vi "PV Pumping station controlling.vi"(8 "error in (no error)":errorcluster, 9 "PV Pumping station - Cluster":T1={"Parameter"=0, "Parameter\nread only<->describe"=FALSE, "Op. mode backing pump"=0, "Pmin for backing-pump\ninterval operations [W]"=40, "Config. Acces. A1 (old version)"=0, "Config. Acces. B1 (old version)"=0, "Pmax for backing-pump\ninterval operations [W]"=40} {"Pmax for backing-pump\ninterval operations [W]" min=30 max=90 step=1; "Config. Acces. B1 (old version)" items=[" fan (constant) (default)", " venting valve", " heating", " backing pump", " fan (temperature controlled)", " seal gas", " always off", " always on"]; "Config. Acces. A1 (old version)" items=[" fan (constant)", " venting valve", " heating", " backing pump", " fan (temperature controlled)", " seal gas", " always off", " always on"]; "Op. mode backing pump" items=[" non-stop", " intermittent", " switch on delayed"]; "Pmin for backing-pump\ninterval operations [W]" min=30 max=90 step=1; "Parameter" items=[" Operations mode backing pump (default)", " Configuration Accessories A1 (old version)", " Configuration Accessories B1 (old version)", " Actual pressure value  [mbar]   (read only)", " Vacuum pressure gauge type", " Pmin for backing-pump interval operations [W]", " Pmax for backing-pump interval operations [W]"]}, 10 "Adress of unit":u16=1 min=1 max=999 step=1, 11 "VISA session":refnum<visa-resource-name>) -> (0 "error out":errorcluster, 2 "response (data)":string, 3 "dup VISA session":refnum<visa-resource-name>)   [LabVIEW 2016, in "Pfeiffer Vacuum.lvlib"]
doc: "There are 7 parameters available, only one of which can be enabled at a time. \n\n0 - Operations mode backing pump (default) (025)\n1 - Configuration Accessories A1 (035)\n (old version - new in PV config A D input output.vi)\n2 - Configuration Accessories B1 (036)\n (old version - new in PV config A D input output.vi)\n3 - Actual pressure value [mbar] (read only) (340)\n4 - Vacuum pressure gauge type (738)\n5 - Pmin for backing-pump interval operations [W] (710)\n6 - Pmax for backing-pump interval operations [W] (711)\n\nNote: Any settings for an parameter that is not selected will be ignored. If a value is out of range, it will be changed to either the upper or the lower limit of the range."
uses:
  Pfeiffer Vacuum.lvlib
  PV Pumping station - Cluster.ctl
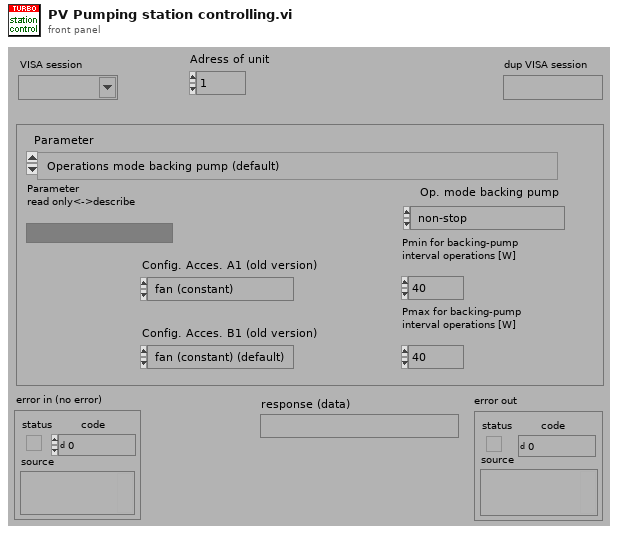
[diagram p1: front panel]
types:
  T1 = typedef "Pfeiffer Vacuum.lvlib/PV Pumping station - Cluster.ctl" = cluster{"Parameter":u16, "Parameter\nread only<->describe":bool, "Op. mode backing pump":u16, "Pmin for backing-pump\ninterval operations [W]":u16, "Config. Acces. A1 (old version)":u16, "Config. Acces. B1 (old version)":u16, "Pmax for backing-pump\ninterval operations [W]":u16}
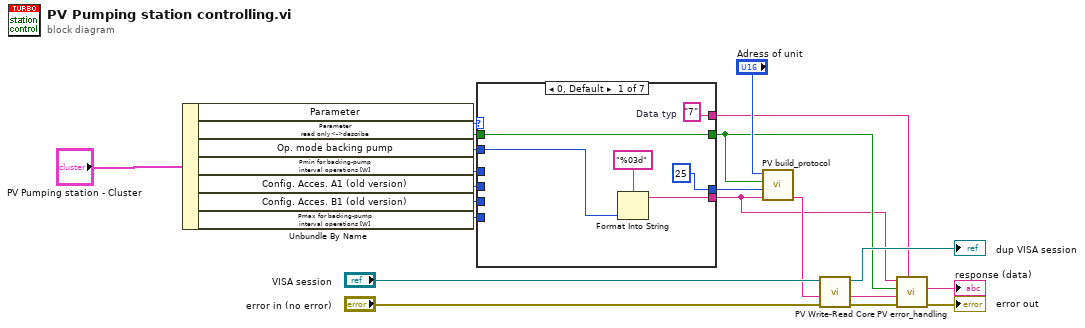
[diagram p0: block diagram]
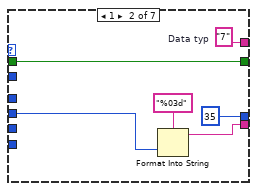
[diagram p2: hidden frame]
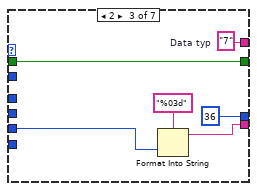
[diagram p3: hidden frame]
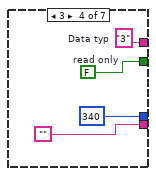
[diagram p4: hidden frame]
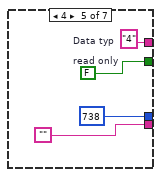
[diagram p5: hidden frame]
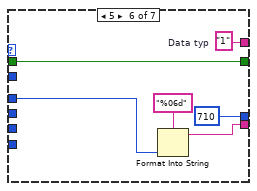
[diagram p6: hidden frame]
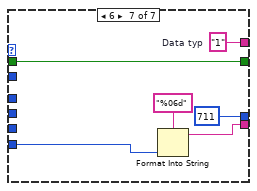
[diagram p7: hidden frame]
diagram:
  n1 = Unbundle By Name("PV Pumping station - Cluster") -> ("Parameter"=w19:u16, "Parameter\nread only<->describe"=w18:bool, "Op. mode backing pump"=w2:u16, "Pmin for backing-pump\ninterval operations [W]"=w14:u16, "Config. Acces. A1 (old version)"=w17:u16, "Config. Acces. B1 (old version)"=w16:u16, "Pmax for backing-pump\ninterval operations [W]"=w15:u16)
  n2 = case shown="0, Default" w19 {
    tunnel: [u16 25 ("Parameter-number") u16 35 ("Parameter-number") u16 36 ("Parameter-number") u16 340 ("Parameter-number") u16 738 ("Parameter-number") u16 710 ("Parameter-number") u16 711 ("Parameter-number")] -> w20
    tunnel: [w22 w31 w37 "" "" w51 w57] -> w6
    tunnel: [w26 w32 w38 w42 w45 w52 w58] -> w7
    tunnel: w18 -> [w26 w32 w38 _ _ w52 w58]
    tunnel: w17 -> [_ w29 _ _ _ _ _]
    tunnel: w16 -> [_ _ w35 _ _ _ _]
    tunnel: w15 -> [_ _ _ _ _ _ w55]
    tunnel: w14 -> [_ _ _ _ _ w49 _]
    tunnel: [w25 w28 w34 w40 w44 w48 w54] -> w5
    tunnel: w2 -> [w23 _ _ _ _ _ _]
    frame 0, Default {
      w25 = "7"  # Data typ
      n3 = Format Into String(format string="%03d" ("Format-String"), w23) -> (resulting string=w22:string)  [unwired: 2 in, 1 out]
    }
    frame 1 {
      w28 = "7"  # Data typ
      n4 = Format Into String(format string="%03d" ("Format-String"), w29) -> (resulting string=w31:string)  [unwired: 2 in, 1 out]
    }
    frame 2 {
      w34 = "7"  # Data typ
      n5 = Format Into String(format string="%03d" ("Format-String"), w35) -> (resulting string=w37:string)  [unwired: 2 in, 1 out]
    }
    frame 3 {
      w40 = "3"  # Data typ
      w42 = FALSE  # read only
    }
    frame 4 {
      w44 = "4"  # Data typ
      w45 = FALSE  # read only
    }
    frame 5 {
      w48 = "1"  # Data typ
      n6 = Format Into String(format string="%06d" ("Format-String"), w49) -> (resulting string=w51:string)  [unwired: 2 in, 1 out]
    }
    frame 6 {
      w54 = "1"  # Data typ
      n7 = Format Into String(format string="%06d" ("Format-String"), w55) -> (resulting string=w57:string)  [unwired: 2 in, 1 out]
    }
  }
  n8 = call "PV build_protocol.vi"("Data"=w6, "Parameter-number"=w20, "parameter\nread<->describe"=w7, "Adress"="Adress of unit") -> ("output"=w11:string)  [unwired: 3 in]
  n9 = call "PV Write-Read Core.vi"("error in"="error in (no error)", "Write data in"=w11, "VISA session"="VISA session") -> ("error out"=w8:errorcluster, "response (data) out"=w9:string, "dup VISA session"=→"dup VISA session":refnum<visa-resource-name>)  [unwired: 2 in]
  n10 = call "PV error_handling.vi"("Data Typ in"=w5, "error in"=w8, "response (data) in"=w9, "Parameter\nread only<->describe"=w7, "data in"=w6) -> ("error out"=→"error out":errorcluster, "Data out"=→"response (data)":string)  [unwired: 4 in, 1 out]
